vi "channel operation tests.vi"() -> ()   [LabVIEW 2014, in "Simple Sequencer TBM tests.lvlib"]
uses:
  <vilib>/NI/TBM Modules/Sequencer/testing/Simple Sequencer TBM tests.lvlib
  <vilib>/NI/TBM Modules/Sequencer/module/configuration/Simple Sequencer TBM configuration.lvclass
panel:
  out "error out":errorcluster
  out "channels match":bool
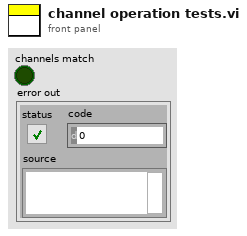
[diagram p1: front panel]
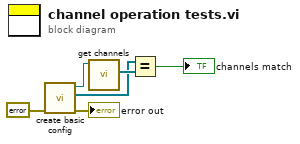
[diagram p0: block diagram]
diagram:
  n1 = call <vilib>:"create basic config.vi"("error in"=errorcluster {"status"=FALSE, "code"=0, "source"=""} ("error out")) -> ("error out"=→"error out":errorcluster, "generated channels"=w4:refnum<class "TBM channel.lvclass">[], "user tag bus module configuration out"=w3:refnum<class "Simple Sequencer TBM configuration.lvclass">)  [unwired: 7 in, 1 out]
  n2 = call-dynamic "get channels.vi"("Simple Sequencer TBM configuration in"=w3) -> ("channels"=w6:refnum<class "TBM channel.lvclass">[])  [unwired: 9 in, 1 out]
  n3 = Equal?(x=w4, y=w6) -> (x = y?=→"channels match":bool)
